vi "BeadCoolerFixedZ(SubVI).vi"(1 "AI0":i16, 2 "Dc Pos":i16, 5 "ig":fxp<+/-,24,6>, 6 "lp coeff":i32[](array[numeric])=[-955995012, 2025731616, 1001305, -1023351008, 2092954700, 1034533], 7 "dg":fxp<+/-,24,12>, 8 "hp coeff":i32[](array[numeric])=[946630756, 1010186290], 9 "pg":fxp<+/-,24,12>, 13 "Upper lim":fxp<+/-,16,16>, 14 "Lower lim":fxp<+/-,16,16>) -> (10 "Output":fxp<+/-,16,16>)   [LabVIEW 2014]
uses:
  <vilib>/rvi/FXPMathLib/basic elements/FxpIntAccumulator/subVIs/nifxpmath_IntAccumulator_SimConfig.ctl
  <vilib>/rvi/FXPMathLib/basic elements/FxpIntAccumulator/simVIs/DllFxpIntAccumulator_sub.vi
  <vilib>/rvi/FXPMathLib/FxpInterpret/XNode/nifxpmath_Interpret.xnode
  <vilib>/rvi/FXPMathLib/basic elements/FxpIntAccumulator/XNode/nifxpmath_IntAccumulator.xnode
  <vilib>/rvi/Analysis/measure/butterworth/XNode/niFpgaButterworthFilter.xnode
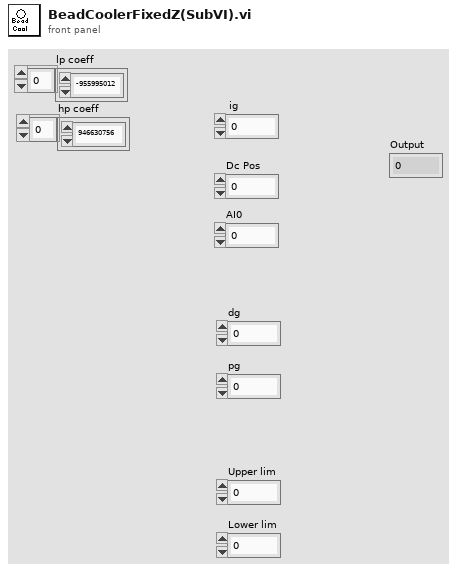
[diagram p1: front panel]
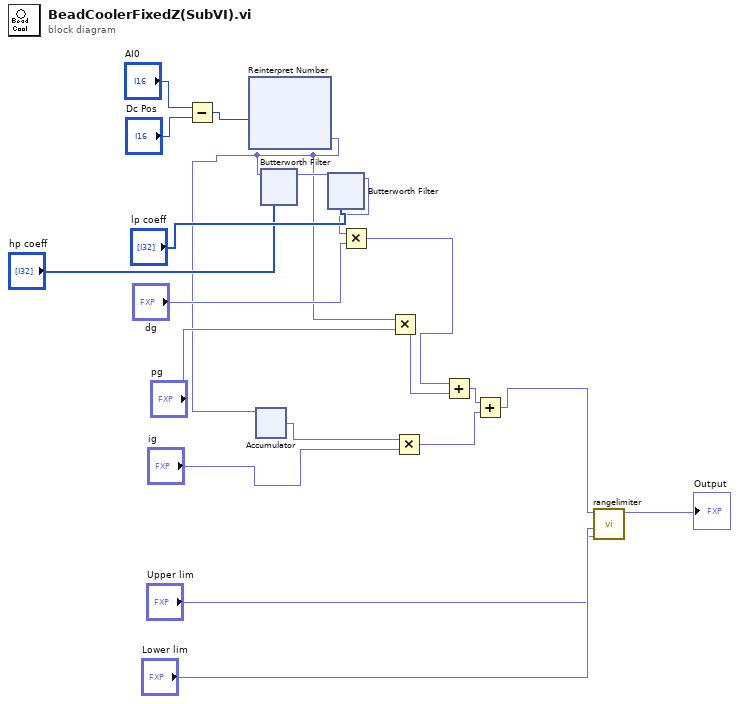
[diagram p0: block diagram]
diagram:
  n1 = Subtract(x="AI0", y="Dc Pos") -> (x-y=w14:i16)
  n2 = xnode "Reinterpret Number"("x"=w14) -> ("y"=w1:fxp<+/-,16,16>)
  n3 = xnode "Accumulator"("x"=w1) -> ("s"=w7:fxp<+/-,32,32>)  [unwired: 4 in, 1 out]
  n4 = xnode "Butterworth Filter"("input data"=w1, "scaled coefficients"="hp coeff") -> ("output data"=w4:fxp<+/-,16,16>)  [unwired: 1 in]
  n5 = xnode "Butterworth Filter"("input data"=w4, "scaled coefficients"="lp coeff") -> ("output data"=w3:fxp<+/-,16,16>)  [unwired: 1 in]
  n6 = Multiply(x=w3, y="dg") -> (x*y=w2:fxp<+/-,18,16>)
  n7 = Multiply(x=w1, y="pg") -> (x*y=w20:fxp<+/-,18,16>)
  n8 = Multiply(x=w7, y="ig") -> (x*y=w9:fxp<+/-,18,16>)
  n9 = Add(x=w2, y=w20) -> (x+y=w11:fxp<+/-,18,16>)
  n10 = Add(x=w11, y=w9) -> (x+y=w10:fxp<+/-,16,16>)
  n11 = call "rangelimiter.vi"("Upper lim"="Upper lim", "Lower lim"="Lower lim", "Input"=w10) -> ("Output"=→"Output":fxp<+/-,16,16>)  [unwired: 8 in]
